vi "Data Acquisition VI.vi"() -> ()   [LabVIEW 2010]
panel:
  out "Waveform Graph":u16[](graph)
  in  "Range":i32(ring)=2 items=["Not Programmable"=0, "+- 20 V"=27, "+- 10 V"=1, "+- 5 V"=2, "+- 4 V"=28, "+- 2.5 V"=3, "+- 2 V"=29, "+- 1.67 V"=4, "+- 1.25 V"=5, "+- 1 V"=6, "+- .625 V"=7, "+- .5 V"=8, "+- .25 V"=30, "+- .2 V"=31, "+- .1 V"=9, "+- .05 V"=10, "+- .01 V"=11, "+- .005 V"=12, "0 - 10 V"=13, "0 - 5 V"=14, "0 - 4 V"=36, "0 - 2.5 V"=15, "0 - 2 V"=16, "0 - 1.67 V"=17, "0 - 1.25 V"=18, "0 - 1 V"=19, "0 - .5 V"=32, "0 - .25 V"=33, "0 - .2 V"=34, "0 - .1 V"=20, "0 - .02 V"=35, "0 - .01 V"=21, "4 - 20 mA"=22, "2 - 10 mA"=23, "1 - 5 mA"=24, ".5 - 2.5 mA"=25, "0 - 20 mA"=26]
  in  "Channel":i32
  in  "BoardNum":u32
  out "Waveform Chart":u16(graph)
  in  "stop":bool
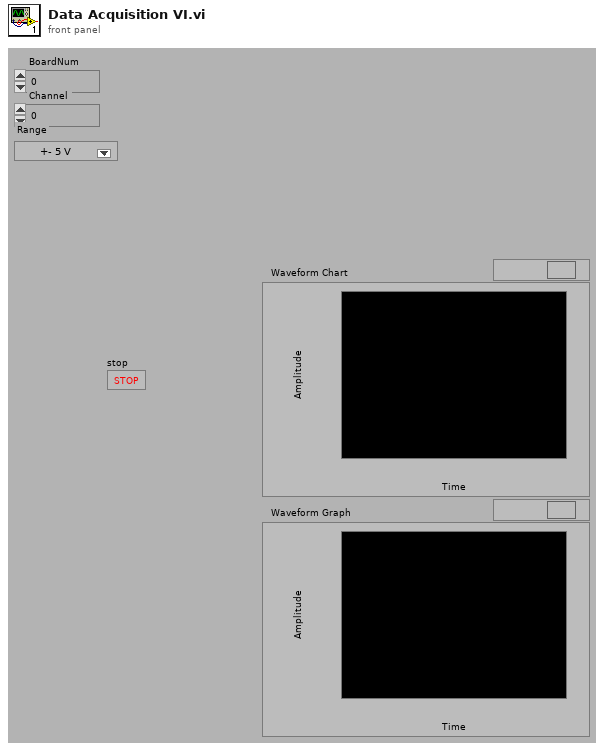
[diagram p1: front panel]
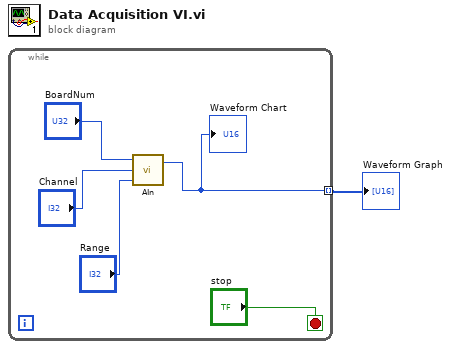
[diagram p0: block diagram]
diagram:
  n1 = while {
    tunnel: [w2] -> w1 mode=indexing
    stop <- "stop" stop-if-true
    n2 = call <menus>:"AIn.VI"("Range"="Range", "Channel"="Channel", "BoardNum"="BoardNum") -> ("DataValue"=w2:u16)  [unwired: 1 out]
    "Waveform Chart" <- w2
  }
  "Waveform Graph" <- w1
